vi "Start_Monitors.vi"() -> ()   [LabVIEW 2015]
uses:
  Instrument_Setup.vi
  Global/Global Variables/global.vi
  Global/Global Variables/Data_Display_global.vi
panel:
  out "Torque":bool
  out "Keithley 2440":bool
  out "Keithley 6221":bool
  out "LS340":bool
  out "Magnet Control":string
  out "AH 2700":bool
  out "LS372":bool
  out "LS370":bool
  out "SR830 Running":bool
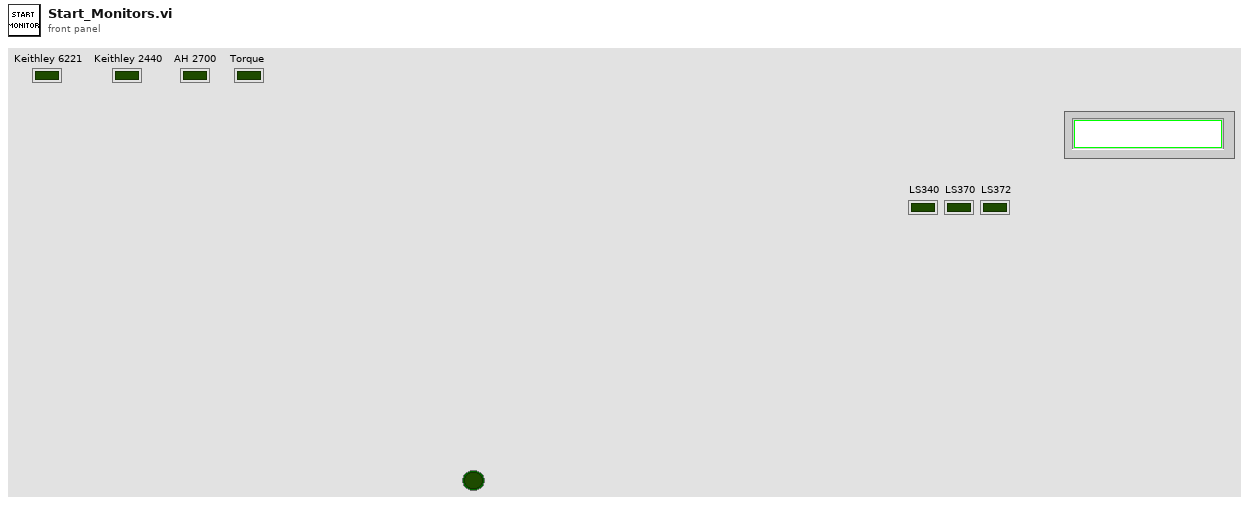
[diagram p1: front panel]
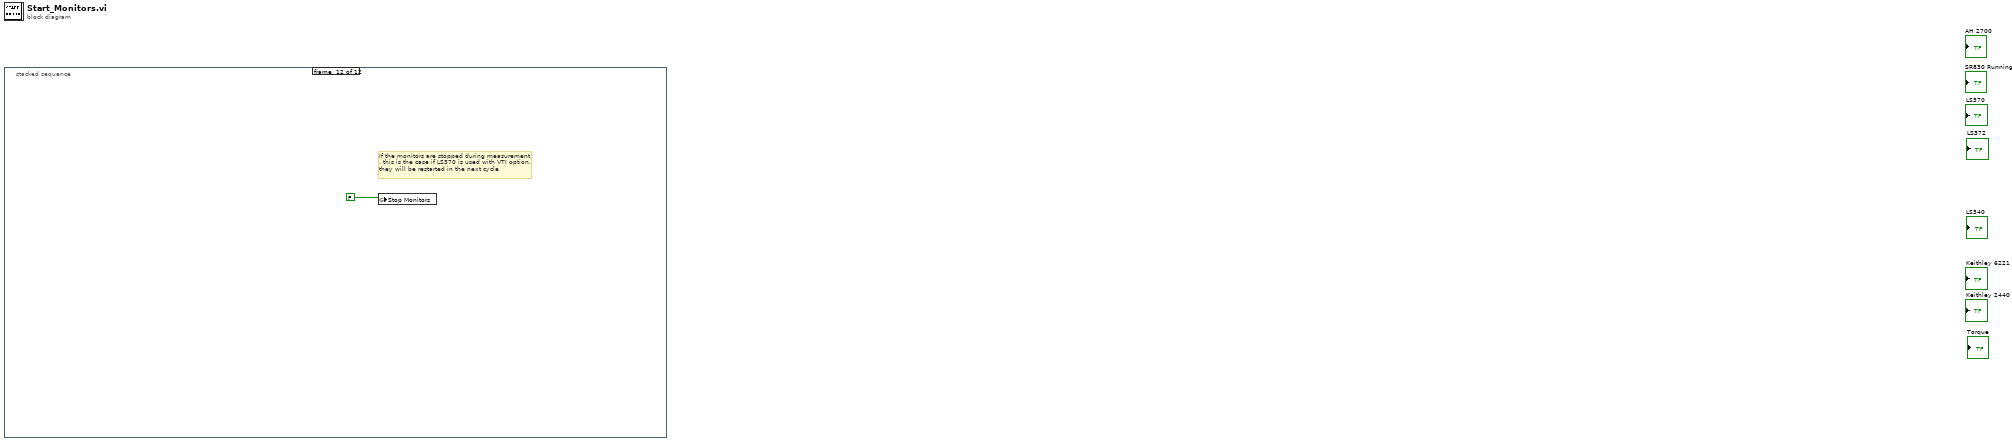
[diagram p0: block diagram]
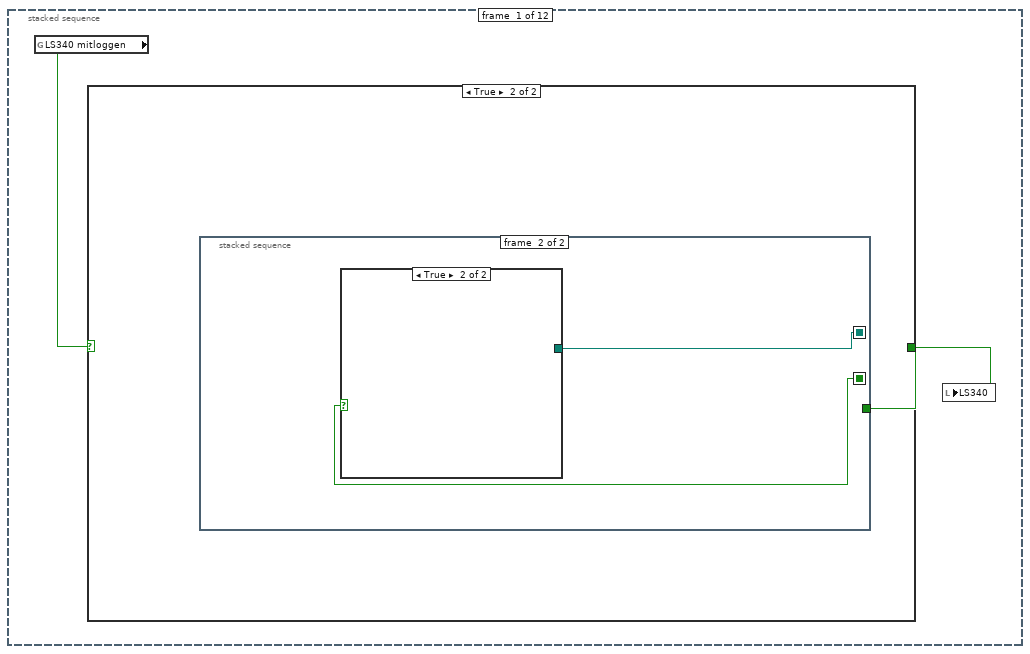
[diagram p2: hidden frame]
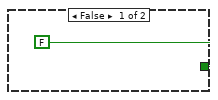
[diagram p3: hidden frame]
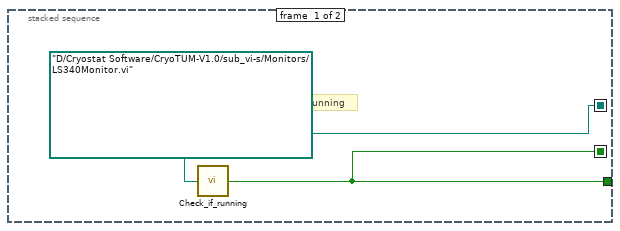
[diagram p4: hidden frame]
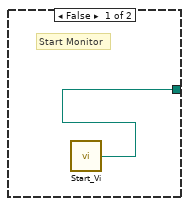
[diagram p5: hidden frame]
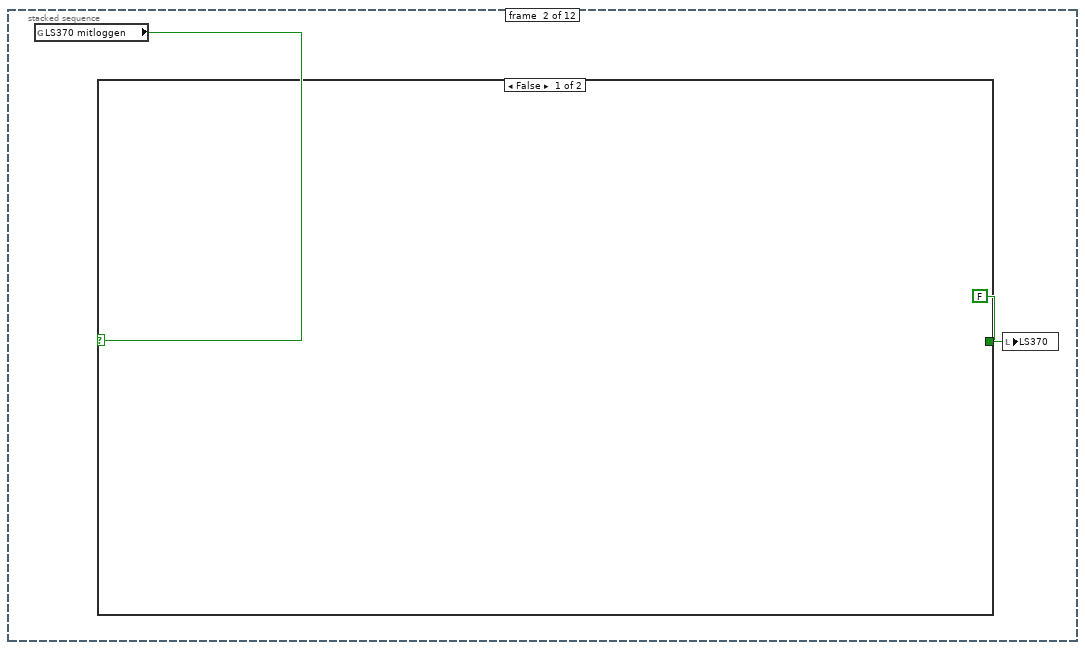
[diagram p6: hidden frame]
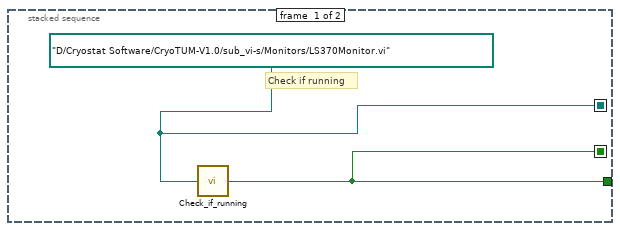
[diagram p8: hidden frame]
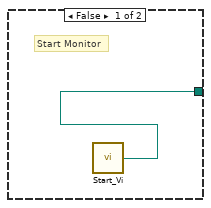
[diagram p9: hidden frame]
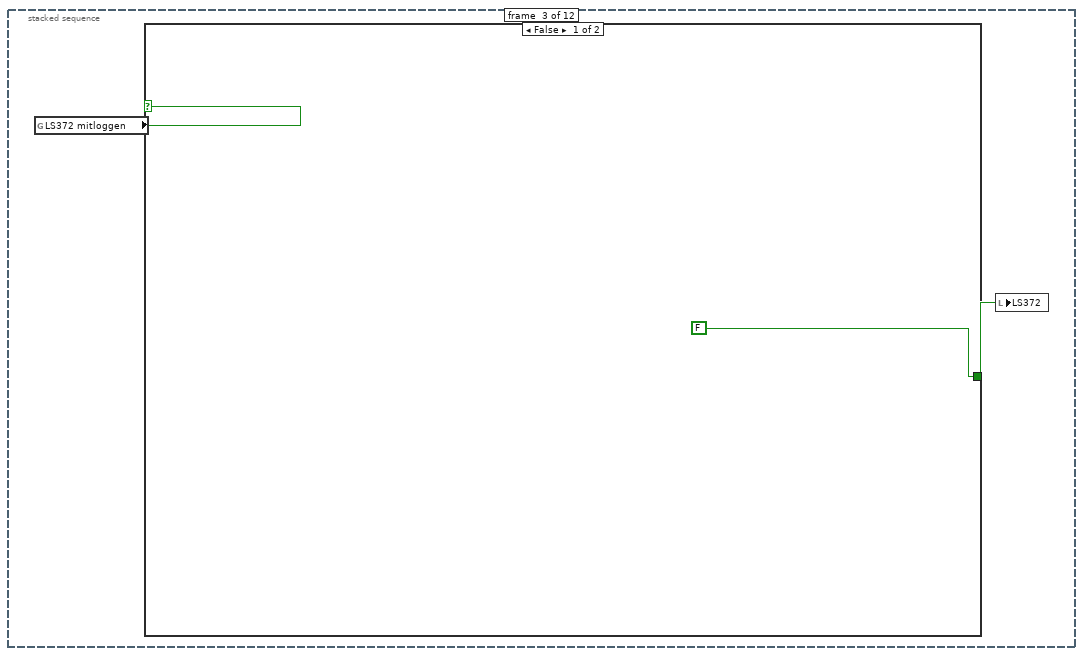
[diagram p10: hidden frame]
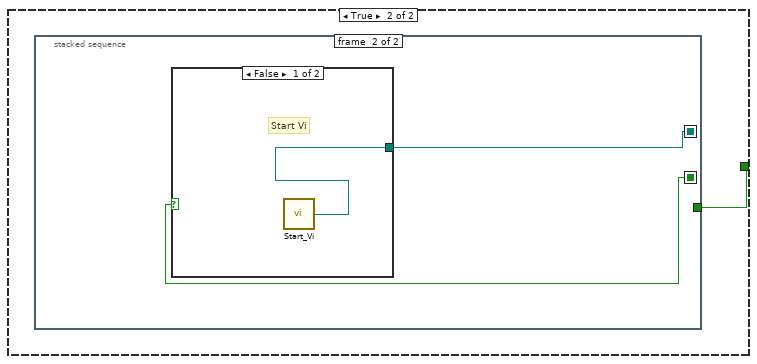
[diagram p11: hidden frame]
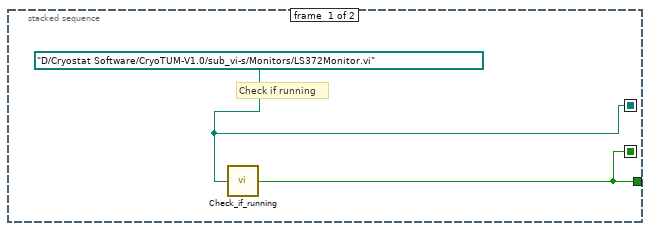
[diagram p12: hidden frame]
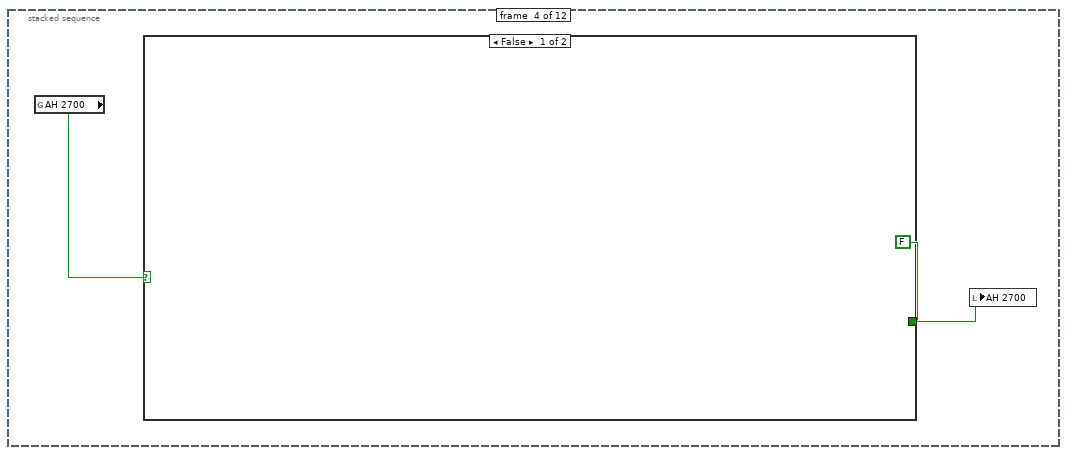
[diagram p14: hidden frame]
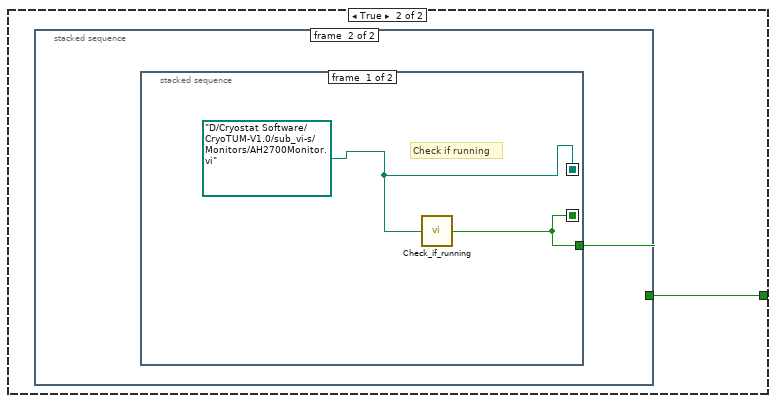
[diagram p15: hidden frame]
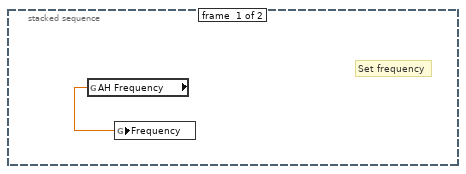
[diagram p16: hidden frame]
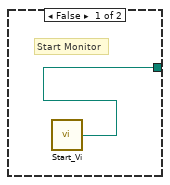
[diagram p18: hidden frame]
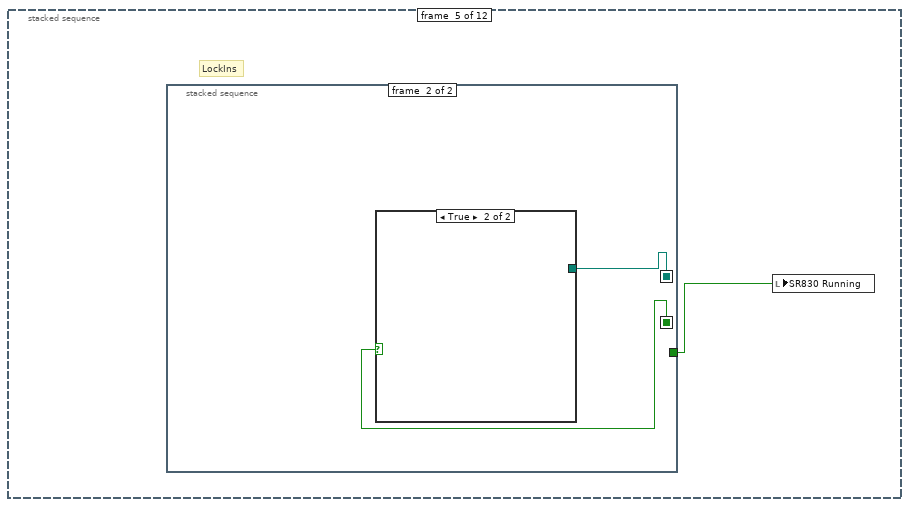
[diagram p19: hidden frame]
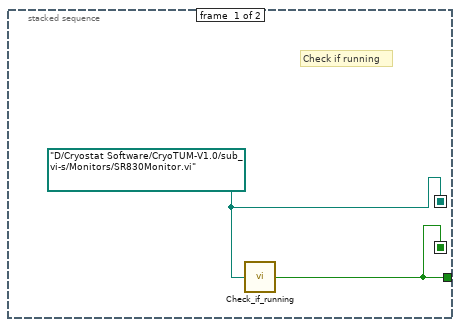
[diagram p20: hidden frame]
diagram:
  n1 = stacked-sequence {
    frame #0 {
      n2 = global read "Instrument_Setup.vi" "LS340 mitloggen"() -> (w2:bool)
      n3 = case shown="True" w2 {
        tunnel: [FALSE w4] -> w1
        frame False {
        }
        frame True {
          n4 = stacked-sequence {
            seq-local: [w5 _] -> [_ w8]
            seq-local: [w6 _] -> [_ w7]
            tunnel: [w6 _] -> w4
            frame #0 {
              w5 = path "D:/Cryostat Software/CryoTUM-V1.0/sub_vi-s/Monitors/LS340Monitor.vi" ("VI-Pfad")
              # "Check if running"
              n5 = call "Check_if_running.vi"("VI-Pfad"=w5) -> ("Running"=w6:bool)
            }
            frame #1 {
              n6 = case shown="True" w7 {
                tunnel: w8 -> [w9 _]
                frame False {
                  # "Start Monitor"
                  n7 = call "Start_Vi.vi"("VI-Pfad"=w9) -> ()  [unwired: 1 in]
                }
                frame True {
                }
              }
            }
          }
        }
      }
      n8 = local write "LS340"(w1) -> ()
    }
    frame #1 {
      n9 = global read "Instrument_Setup.vi" "LS370 mitloggen"() -> (w11:bool)
      n10 = case shown="False" w11 {
        tunnel: [FALSE w13] -> w10
        frame False {
        }
        frame True {
          n11 = stacked-sequence {
            seq-local: [w14 _] -> [_ w17]
            seq-local: [w15 _] -> [_ w16]
            tunnel: [w15 _] -> w13
            frame #0 {
              w14 = path "D:/Cryostat Software/CryoTUM-V1.0/sub_vi-s/Monitors/LS370Monitor.vi" ("VI-Pfad")
              # "Check if running"
              n12 = call "Check_if_running.vi"("VI-Pfad"=w14) -> ("Running"=w15:bool)
            }
            frame #1 {
              n13 = case shown="True" w16 {
                tunnel: w17 -> [w18 _]
                frame False {
                  # "Start Monitor"
                  n14 = call "Start_Vi.vi"("VI-Pfad"=w18) -> ()  [unwired: 1 in]
                }
                frame True {
                }
              }
            }
          }
        }
      }
      n15 = local write "LS370"(w10) -> ()
    }
    frame #2 {
      n16 = global read "Instrument_Setup.vi" "LS372 mitloggen"() -> (w20:bool)
      n17 = case shown="False" w20 {
        tunnel: [FALSE w22] -> w19
        frame False {
        }
        frame True {
          n18 = stacked-sequence {
            seq-local: [w23 _] -> [_ w26]
            seq-local: [w24 _] -> [_ w25]
            tunnel: [w24 _] -> w22
            frame #0 {
              w23 = path "D:/Cryostat Software/CryoTUM-V1.0/sub_vi-s/Monitors/LS372Monitor.vi" ("VI-Pfad")
              # "Check if running"
              n19 = call "Check_if_running.vi"("VI-Pfad"=w23) -> ("Running"=w24:bool)
            }
            frame #1 {
              n20 = case shown="False" w25 {
                tunnel: w26 -> [w27 _]
                frame False {
                  # "Start Vi"
                  n21 = call "Start_Vi.vi"("VI-Pfad"=w27) -> ()  [unwired: 1 in]
                }
                frame True {
                }
              }
            }
          }
        }
      }
      n22 = local write "LS372"(w19) -> ()
    }
    frame #3 {
      n23 = global read "Instrument_Setup.vi" "AH 2700"() -> (w29:bool)
      n24 = case shown="False" w29 {
        tunnel: [FALSE w31] -> w28
        frame False {
        }
        frame True {
          n25 = stacked-sequence {
            tunnel: [_ w33] -> w31
            frame #0 {
              # "Set frequency"
              n26 = global read "Instrument_Setup.vi" "AH Frequency"() -> (w32:dbl)
              n27 = global write "global.vi" "Frequency"(w32) -> ()
            }
            frame #1 {
              n28 = stacked-sequence {
                seq-local: [w34 _] -> [_ w37]
                seq-local: [w35 _] -> [_ w36]
                tunnel: [w35 _] -> w33
                frame #0 {
                  w34 = path "D:/Cryostat Software/CryoTUM-V1.0/sub_vi-s/Monitors/AH2700Monitor.vi" ("VI-Pfad")
                  # "Check if running"
                  n29 = call "Check_if_running.vi"("VI-Pfad"=w34) -> ("Running"=w35:bool)
                }
                frame #1 {
                  n30 = case shown="True" w36 {
                    tunnel: w37 -> [w38 _]
                    frame False {
                      # "Start Monitor"
                      n31 = call "Start_Vi.vi"("VI-Pfad"=w38) -> ()  [unwired: 1 in]
                    }
                    frame True {
                    }
                  }
                }
              }
            }
          }
        }
      }
      n32 = local write "AH 2700"(w28) -> ()
    }
    frame #4 {
      # "LockIns"
      n33 = stacked-sequence {
        seq-local: [w41 _] -> [_ w43]
        seq-local: [w40 _] -> [_ w42]
        tunnel: [w40 _] -> w39
        frame #0 {
          w41 = path "D:/Cryostat Software/CryoTUM-V1.0/sub_vi-s/Monitors/SR830Monitor.vi" ("VI-Pfad")
          # "Check if running"
          n34 = call "Check_if_running.vi"("VI-Pfad"=w41) -> ("Running"=w40:bool)
        }
        frame #1 {
          n35 = case shown="True" w42 {
            tunnel: w43 -> [w44 _]
            frame False {
              # "Start Monitor"
              n36 = call "Start_Vi.vi"("VI-Pfad"=w44) -> ()  [unwired: 1 in]
            }
            frame True {
            }
          }
        }
      }
      n37 = local write "SR830 Running"(w39) -> ()
    }
    frame #5 {
      # "Keithley 4R Monitor"
      n38 = global read "Instrument_Setup.vi" "Keithley 4R"() -> (w45:bool)
      n39 = case shown="False" w45 {
        frame False {
        }
        frame True {
          n40 = stacked-sequence {
            seq-local: [w48 _] -> [_ w50]
            seq-local: [w47 _] -> [_ w49]
            tunnel: [w47 _] -> w46
            frame #0 {
              w48 = path "D:/Cryostat Software/CryoTUM-V1.0/sub_vi-s/Monitors/Keithley4RMonitor" ("VI-Pfad")
              # "Check if running"
              n41 = call "Check_if_running.vi"("VI-Pfad"=w48) -> ("Running"=w47:bool)
            }
            frame #1 {
              n42 = case shown="True" w49 {
                tunnel: w50 -> [w51 _]
                frame False {
                  # "Start Monitor"
                  n43 = call "Start_Vi.vi"("VI-Pfad"=w51) -> ()  [unwired: 1 in]
                }
                frame True {
                }
              }
            }
          }
          n44 = local write "Keithley 2440"(w46) -> ()
        }
      }
    }
    frame #6 {
      n45 = global read "Instrument_Setup.vi" "Keithley"() -> (w52:bool)
      n46 = case shown="False" w52 {
        frame False {
        }
        frame True {
          n47 = stacked-sequence {
            seq-local: [w55 _] -> [_ w57]
            seq-local: [w54 _] -> [_ w56]
            tunnel: [w54 _] -> w53
            frame #0 {
              w55 = path "D:/Cryostat Software/CryoTUM-V1.0/sub_vi-s/Monitors/Keithley_Monitor.vi" ("VI-Pfad")
              # "Check if running"
              n48 = call "Check_if_running.vi"("VI-Pfad"=w55) -> ("Running"=w54:bool)
            }
            frame #1 {
              n49 = case shown="False" w56 {
                tunnel: w57 -> [w58 _]
                frame False {
                  # "Start Monitor"
                  n50 = call "Start_Vi.vi"("VI-Pfad"=w58) -> ()  [unwired: 1 in]
                }
                frame True {
                }
              }
            }
          }
          n51 = local write "Keithley 2440"(w53) -> ()
        }
      }
    }
    frame #7 {
      n52 = global read "Instrument_Setup.vi" "Torque \nMeasurem."() -> (w59:bool)
      n53 = case shown="False" w59 {
        frame False {
        }
        frame True {
          n54 = stacked-sequence {
            seq-local: [w62 _] -> [_ w64]
            seq-local: [w61 _] -> [_ w63]
            tunnel: [w61 _] -> w60
            frame #0 {
              w62 = path "D:/Cryostat Software/CryoTUM-V1.0/sub_vi-s/Monitors/TorqueMotorMonitor.vi" ("VI-Pfad")
              # "Check if running"
              n55 = call "Check_if_running.vi"("VI-Pfad"=w62) -> ("Running"=w61:bool)
            }
            frame #1 {
              n56 = case shown="False" w63 {
                tunnel: w64 -> [w65 _]
                frame False {
                  # "Start Monitor"
                  n57 = call "Start_Vi.vi"("VI-Pfad"=w65) -> ()  [unwired: 1 in]
                }
                frame True {
                }
              }
            }
          }
          n58 = local write "Torque"(w60) -> ()
        }
      }
    }
    frame #8 {
      # "Keithley 6221 so far has no monitor, as no data is collected"
      n59 = global read "Instrument_Setup.vi" "Keithley 6221"() -> (w66:bool)
      n60 = local write "Keithley 6221"(w66) -> ()
    }
    frame #9 {
      # "ILM"
      n61 = stacked-sequence {
        seq-local: [w68 _] -> [_ w70]
        seq-local: [w67 _] -> [_ w69]
        frame #0 {
          w68 = path "D:/Cryostat Software/CryoTUM-V1.0/sub_vi-s/Monitors/ILMMonitor.vi" ("VI-Pfad")
          # "Check if running"
          n62 = call "Check_if_running.vi"("VI-Pfad"=w68) -> ("Running"=w67:bool)
        }
        frame #1 {
          n63 = case shown="True" w69 {
            tunnel: w70 -> [w71 _]
            frame False {
              # "Start Monitor"
              n64 = call "Start_Vi.vi"("VI-Pfad"=w71) -> ()  [unwired: 1 in]
            }
            frame True {
            }
          }
        }
      }
    }
    frame #10 {
      # "B Monitor"
      n65 = global read "Instrument_Setup.vi" "JT option"() -> (w75:bool)
      n66 = case shown="False" w75 {
        frame False {
          n67 = stacked-sequence {
            seq-local: [w84 _] -> [_ w86]
            seq-local: [w83 _] -> [_ w85]
            frame #0 {
              w84 = path "D:/Cryostat Software/CryoTUM-V1.0/sub_vi-s/Monitors/ITCMonitor.vi" ("VI-Pfad")
              # "Check if running"
              n68 = call "Check_if_running.vi"("VI-Pfad"=w84) -> ("Running"=w83:bool)
            }
            frame #1 {
              n69 = case shown="True" w85 {
                tunnel: w86 -> [w87 _]
                frame False {
                  # "Start Monitor"
                  n70 = call "Start_Vi.vi"("VI-Pfad"=w87) -> ()  [unwired: 1 in]
                }
                frame True {
                }
              }
            }
          }
        }
        frame True {
        }
      }
      n71 = stacked-sequence {
        seq-local: [w79 _] -> [_ w81]
        seq-local: [w78 _] -> [_ w80]
        tunnel: [_ w80] -> w74
        frame #0 {
          w79 = path "D:/Cryostat Software/CryoTUM-V1.0/sub_vi-s/Monitors/BMonitor.vi" ("VI-Pfad")
          # "Check if running"
          n72 = call "Check_if_running.vi"("VI-Pfad"=w79) -> ("Running"=w78:bool)
        }
        frame #1 {
          n73 = case shown="True" w80 {
            tunnel: w81 -> [w82 _]
            frame False {
              # "Start Monitor"
              n74 = call "Start_Vi.vi"("VI-Pfad"=w82) -> ()  [unwired: 1 in]
            }
            frame True {
            }
          }
        }
      }
      n75 = case shown="True" w74 {
        tunnel: [16711680 16777215] -> w72
        frame False {
        }
        frame True {
        }
      }
      n76 = property on="Magnet Control" class="Str"("Text.BGColor"=w72, "Text.BG Color"=w72) -> ()  [unwired: 2 in, 2 out]
      "Magnet Control" <- "Magnet Control"
    }
    frame #11 {
      # "If the monitors are stopped during measurement \n, this is the case if LS370 is used with VTI option,\nthey will be restarted in the next cycle"
      n77 = global write "Data_Display_global.vi" "Stop Monitors"(FALSE) -> ()
    }
  }
